vi "coupling_to_string.vi"(11 "Coupling data":cdb[][](array[numeric])) -> (3 "Result string":string)   [LabVIEW 2014]
panel:
  # "Output format conversion for coupling data logging (tab separated).  First two numbers in each row are the relative time and record type, which are dumped as real numbers, the remainder are complex couplings."
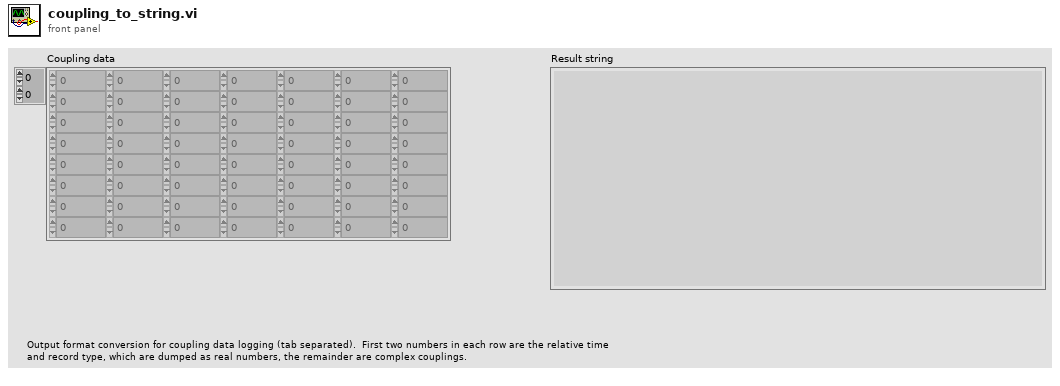
[diagram p1: front panel]
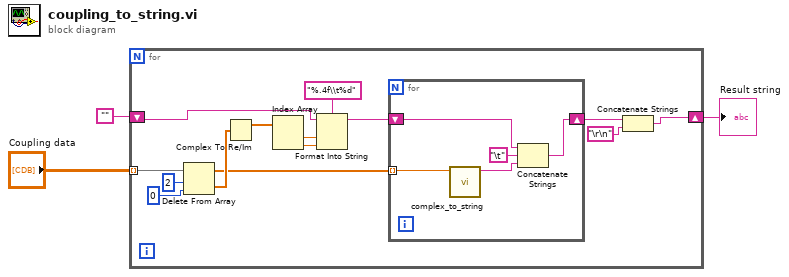
[diagram p0: block diagram]
diagram:
  n1 = for {
    tunnel: "Coupling data" -> [w13] mode=indexing
    shift-right: [w4] -> w1
    shift-left: "" -> [w7]
    n2 = Delete From Array(array=w13, length=2, index=0) -> (deleted portion=w10:cdb[], array with subset deleted=w9:cdb[])
    n3 = Complex To Re/Im(x + iy=w10) -> (x=w16:dbl[])  [unwired: 1 out]
    n4 = Index Array(array=w16) -> (element #1=w15:dbl, element #2=w14:dbl)  [unwired: 2 in]
    n5 = Format Into String(format string="%.4f\\t%d", initial string=w7, w15, w14) -> (resulting string=w8:string)  [unwired: 1 in, 1 out]
    n6 = for {
      tunnel: w9 -> [w22] mode=indexing
      shift-right: [w18] -> w6
      shift-left: w8 -> [w19]
      n7 = call "complex_to_string.vi"("Numeric"=w22) -> ("output string"=w21:string)  [unwired: 10 in]
      n8 = Concatenate Strings(w19, "\t" ("string"), w21) -> (w18:string)
    }
    n9 = Concatenate Strings(w6, "\r\n") -> (w4:string)
  }
  "Result string" <- w1
